vi "WriteToReport.vi"(8 "error in":errorcluster, 10 "Value":string, 11 "Header":T1="Low Pressure Initial") -> (0 "error out":errorcluster)   [LabVIEW 2018, in "S3.lvclass"]
uses:
  S3.lvclass
  Public Controls/ReportHeader.ctl
  Queue/Queue Data.ctl
  Queue/State.ctl
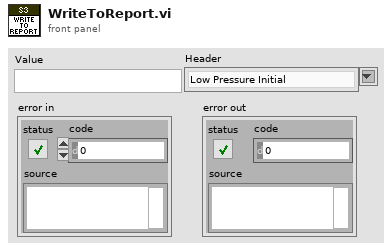
[diagram p1: front panel]
types:
  T1 = typedef "S3.lvclass/ReportHeader.ctl" = string
  T2 = typedef "S3.lvclass/Queue Data.ctl" = cluster{"State":T3, "Data":variant}
  T3 = typedef "S3.lvclass/State.ctl" = enum16{"Initialize", "SetConfig", "AckAlarm", "Alarm", "Idle", "LockLid", "LowPressure", "Pressurize", "DecayTest", "Vent", "Abort", "Start", "CreateReports", "WriteToReport", "WritePressure", "Error", "Exit"}
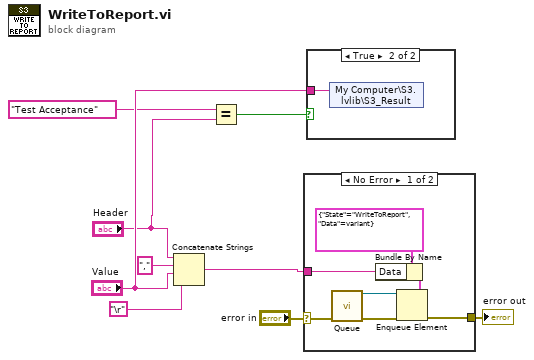
[diagram p0: block diagram]
diagram:
  n1 = Concatenate Strings("Header", "," ("string"), "Value", "\r") -> (w5:string)
  n2 = Equal?(x=T1 "Test Acceptance" ("Header"), y="Header") -> (x = y?=w1:bool)
  n3 = case shown="No Error" "error in" {
    selector: "error in" -> [w16 w17]
    tunnel: [w13 w17] -> w9
    tunnel: w5 -> [w10 _]
    frame No Error {
      n4 = call "Queue.vi"("error in"=w16) -> ("error out"=w15:errorcluster, "queue out"=w14:refnum<queue>)  [unwired: 9 in]
      n5 = Bundle By Name(cluster=T2 {"State"=enum."WriteToReport", "Data"=variant} ("element"), "Data"=w10) -> (w11:T2)
      n6 = Enqueue Element(queue=w14, element=w11, error in (no error)=w15) -> (error out=w13:errorcluster)  [unwired: 1 in, 2 out]
    }
    frame Error {
    }
  }
  "error out" <- w9
  n7 = case shown="True" w1 {
    tunnel: "Value" -> [_ w18]
    frame False {
    }
    frame True {
      n8 = shared-variable "My Computer\\S3.lvlib\\S3_Result"(w18) -> ()  [unwired: 1 in, 1 out]
    }
  }
